vi "DestroyShutdownNotifier.vi"(8 "error in (no error)":errorcluster, 11 "Notifier in":refnum<notifier>) -> ()   [LabVIEW 2013]
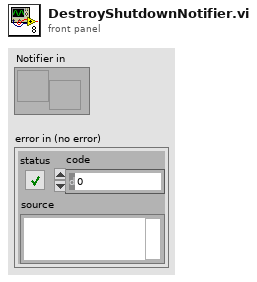
[diagram p1: front panel]
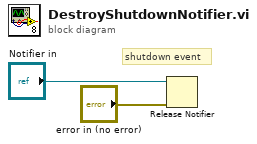
[diagram p0: block diagram]
diagram:
  # "shutdown event"
  n1 = Release Notifier(notifier="Notifier in", error in (no error)="error in (no error)") -> ()  [unwired: 1 in, 3 out]
